vi "Configure Digital Output Frame Polarity.vi"(8 "error in (no error)":errorcluster, 10 "Frame Polarity (0: Positive)":i32(ring) items=["Positive", "Negative"], 11 "VISA resource name":refnum<visa-resource-name>) -> (0 "error out":errorcluster, 3 "VISA resource name out":refnum<visa-resource-name>)   [LabVIEW 2018, in "Agilent PSG MXG Series.lvlib"]
doc: "Configures the polarity of the frame marker for serial transmission. The frame marker indicates the beginning of each sample or byte of data.\n\n<b>Note:</b>\n(1) It is only valid in N5172B/82B with <b>Option 003</b> or <b>Option 004</b> or <b>Option both</b>.\n(2) It is valid for serial transmission only."
uses:
  Agilent PSG MXG Series.lvlib
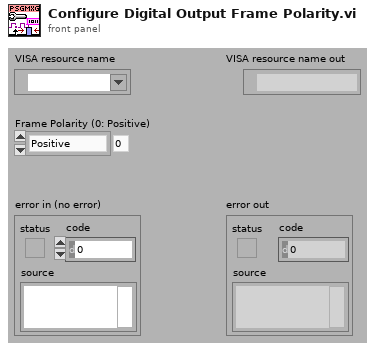
[diagram p1: front panel]
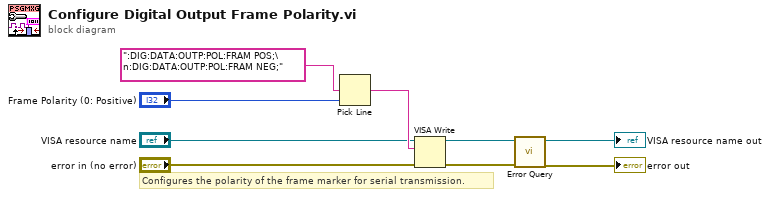
[diagram p0: block diagram]
diagram:
  # "Configures the polarity of the frame marker for serial transmission."
  n1 = Pick Line(multi-line string=":DIG:DATA:OUTP:POL:FRAM POS;\n:DIG:DATA:OUTP:POL:FRAM NEG;", line index="Frame Polarity (0: Positive)") -> (output string=w7:string)  [unwired: 1 in]
  n2 = VISA Write(VISA resource name="VISA resource name", write buffer=w7, error in (no error)="error in (no error)") -> (VISA resource name out=w4:refnum<visa-resource-name>, error out=w3:errorcluster)  [unwired: 1 out]
  n3 = call "Error Query.vi"("error in (no error)"=w3, "VISA resource name"=w4) -> ("error out"=→"error out":errorcluster, "VISA resource name out"=→"VISA resource name out":refnum<visa-resource-name>)  [unwired: 6 in, 2 out]
